vi "Test_Create All Message Queues.vi"(8 "error in (no error)":errorcluster, 10 "DUT":string, 11 "This VI":refnum<vi>) -> (0 "error out":errorcluster, 3 "Message Queues out":T1)   [LabVIEW 2024, in "Test_2.lvlib" / "Test Message Queue.lvlib"]
doc: "This VI creates and initializes all the message queues for your application. If your application requires more than one message queue, right-click the \"Message Queues\" constant above and select Open Type Def. Add the new Message Queue(s) to the type definition, then initialize them in this VI."
uses:
  Test Message Queue.lvlib
  Test_All Message Queues.ctl
  Test_Enqueue Message (Single).vi
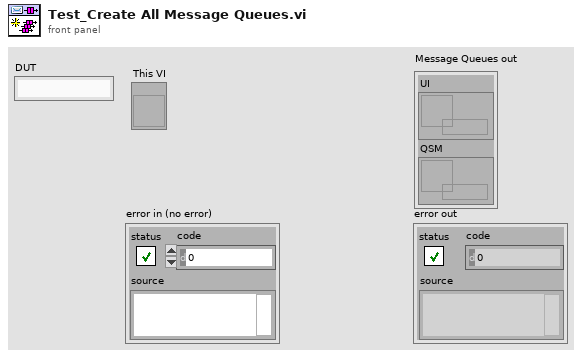
[diagram p1: front panel]
types:
  T1 = typedef "Test_2.lvlib/Test Message Queue.lvlib/Test_All Message Queues.ctl" = cluster{"UI":refnum<queue>, "QSM":refnum<queue>}
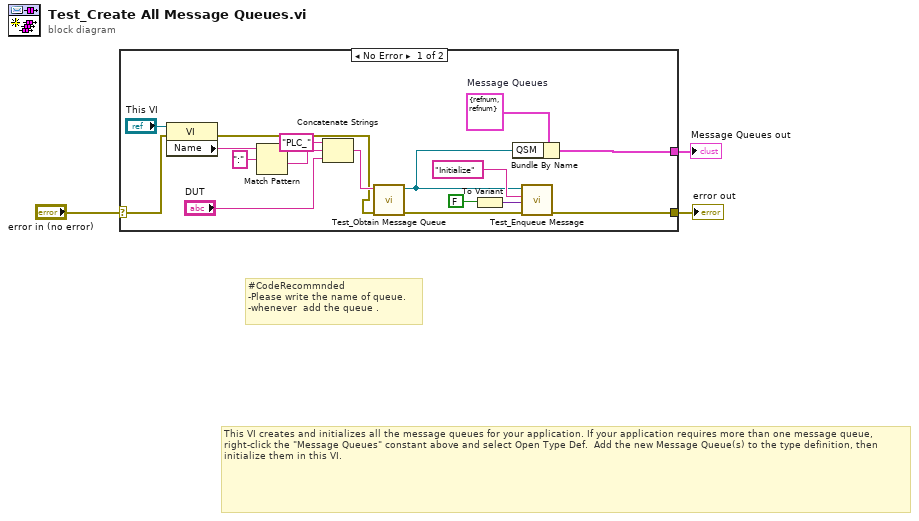
[diagram p0: block diagram]
diagram:
  # "#CodeRecommnded\n-Please write the name of queue.\n-whenever  add the queue ."
  # "This VI creates and initializes all the message queues for your application. If your application requires more than one message queue, right-click the \"Message Queues\" constant above and select Open Type Def.  Add the new Message Queue(s) to the type definition, then initialize them in this VI."
  n1 = case shown="No Error" "error in (no error)" {
    selector: "error in (no error)" -> [w12 w21]
    tunnel: [w20 w21] -> w3
    tunnel: [w18 _] -> w2
    frame No Error {
      w19 = T1 {"UI"=refnum, "QSM"=refnum}  # Message Queues
      n2 = property class="VI"(reference="This VI", error in=w12) -> (error out=w11:errorcluster, "Name"=w9:string)  [unwired: 1 out]
      n3 = Match Pattern(string=w9, regular expression=":") -> (after substring=w7:string)  [unwired: 1 in, 3 out]
      n4 = Concatenate Strings("PLC_" ("string"), w7, "DUT") -> (w14:string)
      n5 = call "Test_Obtain Message Queue.vi"("error in (no error)"=w11, "Queue Name"=w14) -> ("error out"=w17:errorcluster, "Message Queue"=w15:refnum<queue>)  [unwired: 8 in]
      n6 = To Variant(anything=FALSE) -> (Variant=w5:variant)
      n7 = Bundle By Name(cluster=w19, "QSM"=w15) -> (w18:T1)
      n8 = call-poly "Test_Enqueue Message.vi"("error in (no error)"=w17, "Message Data"=w5, "Message"="Initialize", "Message Queue"=w15) -> ("error out"=w20:errorcluster)  [unwired: 6 in, 1 out]
    }
    frame Error {
    }
  }
  "Message Queues out" <- w2
  "error out" <- w3
